vi "Pulsed Experiment.vi"(0 "Optimize Parameters":T3={"Volt Step"={"X"=0.01, "Y"=0.01, "Z"=0.0}, "Num Iterations"=1, "Dwell Time (ms)"=100, "Volts Range"={"X"=0.1, "Y"=0.1, "Z"=0.0}, "Method"={"X"=enum."Max", "Y"=enum."Max", "Z"=enum."Max"}} {"Volts Range"."Z" min=0.0; "Volts Range"."Y" min=0.0; "Volts Range"."X" min=0.0; "Dwell Time (ms)" min=0; "Num Iterations" min=1 step=1; "Volt Step"."Z" min=1e-05; "Volt Step"."Y" min=1e-06; "Volt Step"."X" min=1e-06}, 3 "Contrast XY Graph Refnum":refnum<vi>, 4 "Experiment":T1=enum."Rabi", 5 "# samples":i32, 7 "# time points":i32, 9 "min time":dbl, 10 "Last counts/s ref":refnum<vi>, 11 "max time":dbl, 12 "# scan iterations":i32, 13 "Window Parameters":string, 14 "Save Contrast Options":T2={"Save contrast graph"=FALSE, "Path for contrast graph"=path "C:/experiment/data/may_15_2012/SIL1_NV1_pippin_uW_off", "Save contrast data"=FALSE, "Path for contrast data"=path "C:/experiment/data/may_15_2012/SIL1_NV1_pippin_uW_off"}, 15 "scans done ref":refnum<vi>) -> ()   [LabVIEW 2012]
uses:
  Strict Type Def - Optimize Parameters Cluster.ctl
  SaveContrastOptions.ctl
  States.ctl
  <vilib>/DAQmx/read.llb/DAQmx Read (Counter 1D U32 1Chan NSamp).vi
  Channels.vi
  <vilib>/DAQmx/miscellaneous.llb/DAQmx Fill In Error Info.vi
  Global Vars.vi
  <vilib>/Utility/file.llb/Write To Spreadsheet File (DBL).vi
panel:
  out "Last counts/s":u32
  out "scans done":u32
  out "Readout counts":cluster{"Y":dbl[], "Y":dbl[]}[](graph)
  out "Reference counts":cluster{"Y":dbl[], "Y":dbl[]}[](graph)
  out "Normalized contrast":cluster{"Y":dbl[], "Y":dbl[]}[](graph)
  # "Pulsed Experiments: \nData collection and processing\nRabi\nSpin Echo\nCPMG\nXY-4\n\n08/27/2013, Srujan Meesala\n6/9/2014, Samuel Kim"
  # "Default PB connections:\nPB0 - MW switch\nPB1 - unused\nPB2 - Counter sample clk\nPB3 - Green AOM"
  # "Pulse sequence parameters"
  # "to spreadsheet"
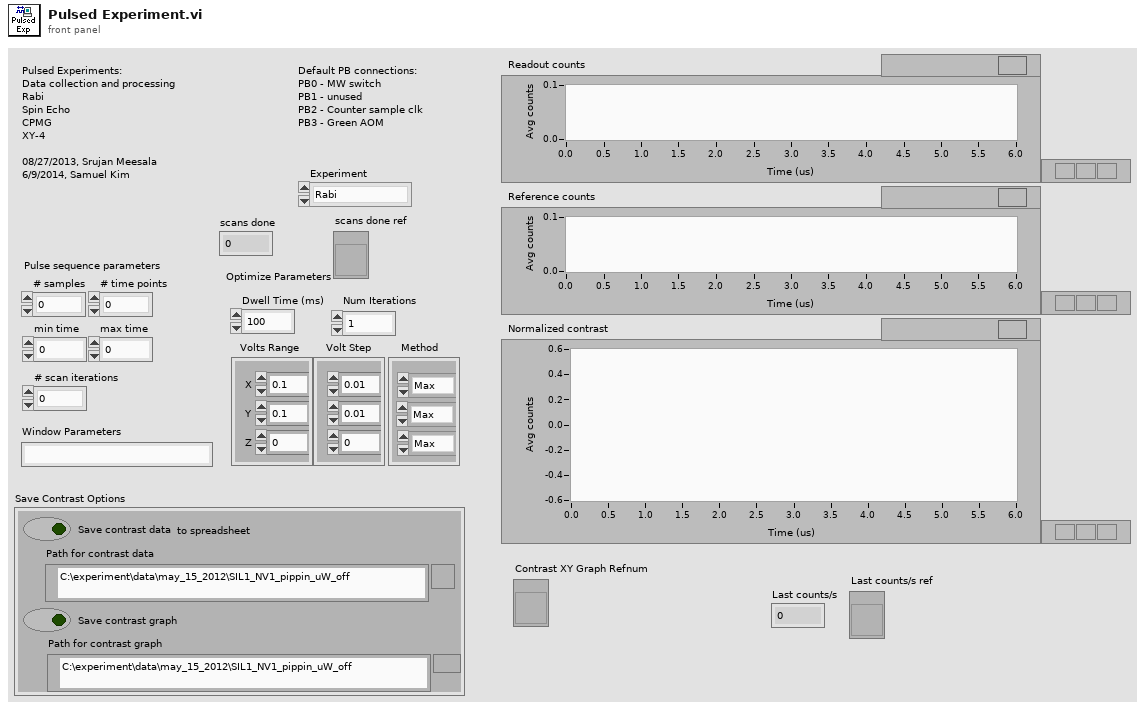
[diagram p1: front panel]
types:
  T1 = typedef "States.ctl" = enum16{"Initialize", "Scan", "Count", "Optimize", "Hold", "ESR", "ESR 2", "Rabi", "Spin Echo", "Spectrum", "Stability", "CPMG", "XY-4", "Exit"}
  T2 = typedef "SaveContrastOptions.ctl" = cluster{"Save contrast graph":bool, "Path for contrast graph":path, "Save contrast data":bool, "Path for contrast data":path}
  T3 = typedef "Strict Type Def - Optimize Parameters Cluster.ctl" = cluster{"Volt Step":cluster{"X":dbl, "Y":dbl, "Z":dbl}, "Num Iterations":i32, "Dwell Time (ms)":i32, "Volts Range":cluster{"X":dbl, "Y":dbl, "Z":dbl}, "Method":cluster{"X":enum16{"Max", "Gaussian"}, "Y":enum16{"Max", "Gaussian"}, "Z":enum16{"Max", "Gaussian"}}}
  T4 = typedef "imagedata.ctl" = cluster{"image type":i32, "image depth":i32, "image":u8[], "mask":u8[], "colors":u32[], "Rectangle":cluster{"left":i16, "top":i16, "right":i16, "bottom":i16}}
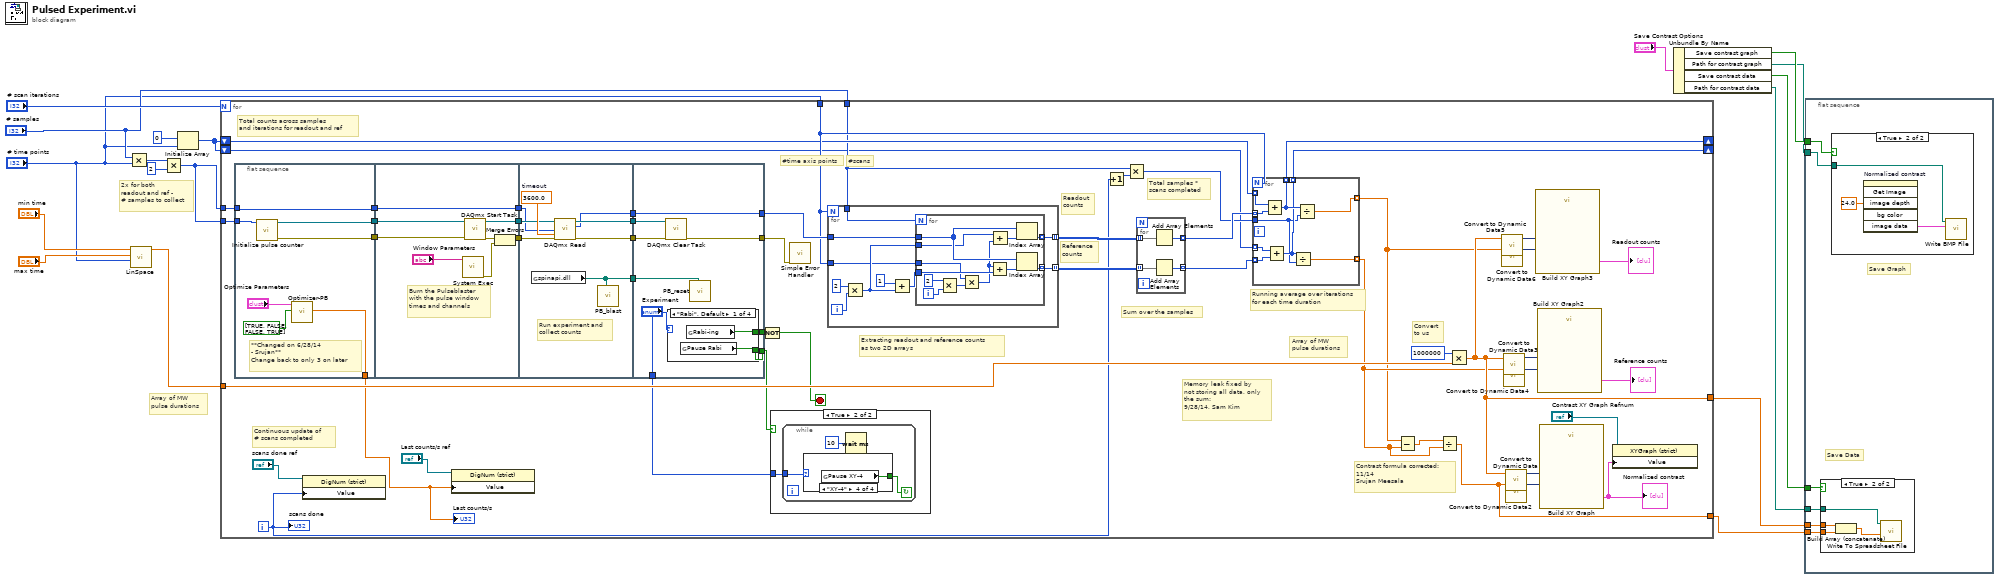
[diagram p0: block diagram]
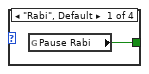
[diagram p5: hidden frame]
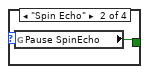
[diagram p6: hidden frame]
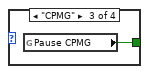
[diagram p7: hidden frame]
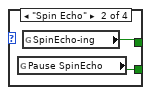
[diagram p8: hidden frame]
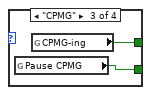
[diagram p9: hidden frame]
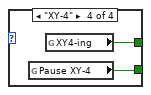
[diagram p10: hidden frame]
diagram:
  # "Array of MW\npulse durations"
  # "2x for both\nreadout and ref -\n# samples to collect"
  n1 = Multiply(x="# samples", y="# time points") -> (x*y=w16:i32)
  n2 = call "LinSpace.vi"("Num Steps"="# time points", "Max"="max time", "Min"="min time") -> ("Array"=w12:dbl[])  [unwired: 8 in]
  n3 = Multiply(x=w16, y=u32 2 ("Reset Count")) -> (x*y=w14:u32)
  n4 = Initialize Array(u32 0 ("Reset Count"), "# time points") -> (w1:u32[])
  n5 = for {
    N: "# scan iterations" -> [_]
    tunnel: [w53] -> w18
    tunnel: [w51] -> w17
    tunnel: w14 -> [w50]
    tunnel: "# samples" -> [w30]
    tunnel: "# time points" -> [w49]
    tunnel: w14 -> [w48]
    shift-right: [w28] -> _
    shift-left: w1 -> [w34]
    shift-right: [w25] -> _
    shift-left: w1 -> [w27]
    tunnel: w12 -> [w41]
    i -> [w22]
    stop <- w38 stop-if-true
    # "Total samples * \nscans completed"
    # "Memory leak fixed by\nnot storing all data, only\nthe sum:\n9/28/14, Sam Kim"
    # "Total counts across samples\nand iterations for readout and ref"
    # "Sum over the samples"
    # "Continuous update of \n# scans completed"
    # "Convert\nto us"
    # "Contrast formula corrected:\n11/14\nSrujan Meesala"
    # "#time axis points"
    # "#scans"
    # "Reference\ncounts"
    # "Readout\ncounts"
    # "Running average over iterations\nfor each time duration"
    # "Array of MW\npulse durations"
    # "Extracting readout and reference counts\nas two 2D arrays"
    n6 = flat-sequence {
      tunnel: w50 -> [w88]
      tunnel: [w88] -> w69
      tunnel: w48 -> [w86]
      tunnel: [w85] -> w47
      tunnel: [w84] -> w46
      tunnel: [w82] -> w19
      tunnel: [w96] -> w68
      tunnel: [w95] -> w67
      tunnel: w69 -> [w95]
      tunnel: w47 -> [w94]
      tunnel: w46 -> [w93]
      tunnel: [w90] -> w40
      tunnel: w68 -> [w103]
      tunnel: [w99] -> w66
      tunnel: [w101] -> w65
      tunnel: [w100] -> w64
      tunnel: w67 -> [w98]
      tunnel: [w97] -> w63
      tunnel: w40 -> [w102]
      tunnel: [w112] -> w61
      tunnel: w66 -> [w112]
      tunnel: w65 -> [w111]
      tunnel: w64 -> [w109]
      tunnel: [w108] -> w62
      tunnel: w63 -> [w110]
      tunnel: [w107] -> w39
      tunnel: [w106] -> w37
      tunnel: ["Experiment"] -> w36
      frame #0 {
        # "**Changed on 6/28/14\n- Srujan**\nChange back to only 3 on later"
        n7 = call "Initialize pulse counter.vi"("Samples per channel"=w86) -> ("error out"=w84:errorcluster, "DAQmx Task Name"=w85:refnum<k21>)  [unwired: 9 in]
        n8 = call "Optimizer-PB.vi"("Optimize active channels"=bool[] [TRUE, FALSE, FALSE, TRUE], "Optimize Parameters"="Optimize Parameters") -> ("Final Counts/s"=w82:dbl)  [unwired: 8 in, 1 out]
      }
      frame #1 {
        # "Burn the Pulseblaster\nwith the pulse window\ntimes and channels"
        n9 = call <vilib>:"System Exec.vi"("command line"="Window Parameters") -> ("error out"=w92:errorcluster)  [unwired: 7 in, 3 out]
        n10 = call <vilib>:"DAQmx Start Task.vi"("task/channels in"=w94, "error in"=w93) -> ("task out"=w96:refnum<k21>, "error out"=w91:errorcluster)  [unwired: 12 in]
        n11 = Merge Errors(w91, w92) -> (w90:errorcluster)
      }
      frame #2 {
        w104 = 3600.0  # timeout
        # "Run experiment and\ncollect counts"
        n12 = global read "Channels.vi" "spinapi.dll"() -> (w97:path)
        n13 = call-poly <vilib>:"DAQmx Read.vi"("task/channels in"=w103, "number of samples per channel"=w98, "timeout"=w104, "error in"=w102) -> ("task out"=w100:refnum<k21>, "data"=w99:u32[], "error out"=w101:errorcluster)  [unwired: 9 in]
        n14 = call "PB_blast.vi"("Path to spinapi.dll"=w97) -> ()  [unwired: 7 in]
      }
      frame #3 {
        n15 = call <vilib>:"DAQmx Clear Task.vi"("task in"=w109, "error in"=w111) -> ("error out"=w108:errorcluster)  [unwired: 13 in]
        n16 = case shown="\"Rabi\", Default" "Experiment" {
          tunnel: [w114 w116 w118 w120] -> w107
          tunnel: [w113 w115 w117 w119] -> w106
          frame "Rabi", Default {
            n17 = global read "Global Vars.vi" "Pause Rabi"() -> (w113:bool)
            n18 = global read "Global Vars.vi" "Rabi-ing"() -> (w114:bool)
          }
          frame "Spin Echo" {
            n19 = global read "Global Vars.vi" "Pause SpinEcho"() -> (w115:bool)
            n20 = global read "Global Vars.vi" "SpinEcho-ing"() -> (w116:bool)
          }
          frame "CPMG" {
            n21 = global read "Global Vars.vi" "Pause CPMG"() -> (w117:bool)
            n22 = global read "Global Vars.vi" "CPMG-ing"() -> (w118:bool)
          }
          frame "XY-4" {
            n23 = global read "Global Vars.vi" "Pause XY-4"() -> (w119:bool)
            n24 = global read "Global Vars.vi" "XY4-ing"() -> (w120:bool)
          }
        }
        n25 = call "PB_reset.vi"("Path to spinapi.dll"=w110) -> ()  [unwired: 7 in]
      }
    }
    n26 = property class="DigNum (strict)"(reference="scans done ref", "Value"=w22) -> ()  [unwired: 1 in, 2 out]
    n27 = property class="DigNum (strict)"(reference="Last counts/s ref", "Value"=w19) -> ()  [unwired: 1 in, 2 out]
    n28 = Not(x=w39) -> (.not. x?=w38:bool)
    n29 = case shown="True" w37 {
      tunnel: w36 -> [_ w74]
      frame False {
      }
      frame True {
        n30 = while {
          tunnel: w74 -> [w75]
          stop <- w76 continue-if-true
          n31 = case shown="\"XY-4\"" w75 {
            tunnel: [w78 w79 w80 w81] -> w76
            frame "Rabi", Default {
              n32 = global read "Global Vars.vi" "Pause Rabi"() -> (w78:bool)
            }
            frame "Spin Echo" {
              n33 = global read "Global Vars.vi" "Pause SpinEcho"() -> (w79:bool)
            }
            frame "CPMG" {
              n34 = global read "Global Vars.vi" "Pause CPMG"() -> (w80:bool)
            }
            frame "XY-4" {
              n35 = global read "Global Vars.vi" "Pause XY-4"() -> (w81:bool)
            }
          }
          n36 = Wait (ms)(milliseconds to wait=u32 10) -> ()  [unwired: 1 out]
        }
      }
    }
    n37 = call <vilib>:"Simple Error Handler.vi"("error in (no error)"=w62) -> ()  [unwired: 4 in, 5 out]
    n38 = for {
      N: w49 -> [_]
      tunnel: w30 -> [w138]
      tunnel: w61 -> [w139]
      tunnel: [w137] -> w33 mode=indexing
      tunnel: [w136] -> w32 mode=indexing
      tunnel: w49 -> [w130]
      i -> [w135]
      n39 = Multiply(x=u32 2 ("Reset Count"), y=w135) -> (x*y=w132:u32)
      n40 = Add(x=u32 1 ("Reset Count"), y=w132) -> (x+y=w131:u32)
      n41 = for {
        N: w138 -> [_]
        tunnel: w139 -> [w151]
        tunnel: [w148] -> w137 mode=indexing
        tunnel: [w147] -> w136 mode=indexing
        tunnel: w132 -> [w146]
        tunnel: w131 -> [w145]
        tunnel: w130 -> [w141]
        i -> [w143]
        n42 = Multiply(x=u32 2 ("Reset Count"), y=w143) -> (x*y=w142:u32)
        n43 = Multiply(x=w141, y=w142) -> (x*y=w140:u32)
        n44 = Add(x=w140, y=w145) -> (x+y=w149:u32)
        n45 = Add(x=w146, y=w140) -> (x+y=w150:u32)
        n46 = Index Array(array=w151, index=w150) -> (element=w148:u32)
        n47 = Index Array(array=w151, index=w149) -> (element=w147:u32)
      }
    }
    n48 = Increment(x=w22) -> (x+1=w21:i32)
    n49 = Multiply(x=w30, y=w21) -> (x*y=w29:i32)
    n50 = for {
      tunnel: w33 -> [w70] mode=indexing
      tunnel: w32 -> [w73] mode=indexing
      tunnel: [w72] -> w31 mode=indexing
      tunnel: [w71] -> w26 mode=indexing
      n51 = Add Array Elements(numeric array=w70) -> (sum=w72:u32)
      n52 = Add Array Elements(numeric array=w73) -> (sum=w71:u32)
    }
    n53 = for {
      N: w49 -> [_]
      tunnel: w34 -> [w128] mode=indexing
      tunnel: [w127] -> w23 mode=indexing
      tunnel: w31 -> [w129] mode=indexing
      tunnel: w29 -> [w122]
      tunnel: [w126] -> w28 mode=indexing
      tunnel: w27 -> [w125] mode=indexing
      tunnel: w26 -> [w124] mode=indexing
      tunnel: [w123] -> w25 mode=indexing
      tunnel: [w121] -> w24 mode=indexing
      n54 = Add(x=w128, y=w129) -> (x+y=w126:u32)
      n55 = Add(x=w125, y=w124) -> (x+y=w123:u32)
      n56 = Divide(x=w123, y=w122) -> (x/y=w121:dbl)
      n57 = Divide(x=w126, y=w122) -> (x/y=w127:dbl)
    }
    n58 = Subtract(x=w23, y=w24) -> (x-y=w52:dbl[])
    n59 = Divide(x=w52, y=w24) -> (x/y=w53:dbl[])
    n60 = Multiply(x=u32 1000000 ("Reset Count"), y=w41) -> (x*y=w51:dbl[])
    n61 = call "Convert to Dynamic Data5"("Array"=w51) -> ("Dynamic Data Type"=w55:dynamicdata)  [unwired: 3 in]
    n62 = call "Convert to Dynamic Data6"("Array"=w23) -> ("Dynamic Data Type"=w54:dynamicdata)  [unwired: 3 in]
    n63 = call "Convert to Dynamic Data3"("Array"=w51) -> ("Dynamic Data Type"=w58:dynamicdata)  [unwired: 3 in]
    n64 = call "Convert to Dynamic Data4"("Array"=w24) -> ("Dynamic Data Type"=w57:dynamicdata)  [unwired: 3 in]
    n65 = call "Convert to Dynamic Data"("Array"=w51) -> ("Dynamic Data Type"=w60:dynamicdata)  [unwired: 3 in]
    n66 = call "Convert to Dynamic Data2"("Array"=w53) -> ("Dynamic Data Type"=w59:dynamicdata)  [unwired: 3 in]
    n67 = call "Build XY Graph3"("Y Input"=w54, "X Input"=w55) -> ("XY Graph"=→"Readout counts":cluster{"Y":dbl[], "Y":dbl[]}[])  [unwired: 3 in, 6 out]
    n68 = call "Build XY Graph2"("Y Input"=w57, "X Input"=w58) -> ("XY Graph"=→"Reference counts":cluster{"Y":dbl[], "Y":dbl[]}[])  [unwired: 3 in, 6 out]
    n69 = call "Build XY Graph"("Y Input"=w59, "X Input"=w60) -> ("XY Graph"=w42:cluster{"Y":dbl[], "Y":dbl[]}[])  [unwired: 3 in, 6 out]
    "Normalized contrast" <- w42
    n70 = property class="XYGraph (strict)"(reference="Contrast XY Graph Refnum", "Value"=w42) -> ()  [unwired: 1 in, 2 out]
    "scans done" <- w22
    "Last counts/s" <- w19
  }
  n71 = Unbundle By Name("Save Contrast Options") -> ("Save contrast graph"=w7:bool, "Path for contrast graph"=w5:path, "Save contrast data"=w6:bool, "Path for contrast data"=w4:path)
  n72 = flat-sequence {
    tunnel: w18 -> [w157]
    tunnel: w17 -> [w156]
    tunnel: w7 -> [w155]
    tunnel: w6 -> [w154]
    tunnel: w5 -> [w153]
    tunnel: w4 -> [w152]
    frame #0 {
      # "Save Graph"
      # "Save Data"
      n73 = case shown="True" w154 {
        tunnel: w156 -> [_ w160]
        tunnel: w157 -> [_ w161]
        tunnel: w152 -> [_ w159]
        frame False {
        }
        frame True {
          n74 = Build Array (concatenate)(w160, w161) -> (w158:dbl[])
          n75 = call-poly <vilib>:"Write To Spreadsheet File.vi"("1D data"=w158, "file path (dialog if empty)"=w159) -> ()  [unwired: 6 in, 1 out]
        }
      }
      n76 = case shown="True" w155 {
        tunnel: w153 -> [_ w162]
        frame False {
        }
        frame True {
          n77 = invoke on="Normalized contrast" class="XYGraph (strict)" method="Get Image"("image depth"=24.0 ("Initial Delay")) -> ("image data"=w163:T4)  [unwired: 5 in, 5 out]
          n78 = call <vilib>:"Write BMP File.vi"("image data"=w163, "path to BMP file"=w162) -> ()  [unwired: 8 in, 2 out]
        }
      }
    }
  }
